vi "iRobot UART Read.vi"(8 "error in":errorcluster, 9 "timeout (ms)":i32=-1, 10 "Number of Bytes":u32, 11 "UART port in":T1) -> (0 "error out":errorcluster, 1 "UART Stream":u8[](array[numeric]), 2 "Timed Out?":bool, 3 "UART port out":T1)   [LabVIEW 2015]
doc: "Read data from the UART receive buffer until <b>Number of Bytes</b> have been received, or until a timeout occurs. A negative timeout means wait indefinitely."
uses:
  iRobot UART Port Type.ctl
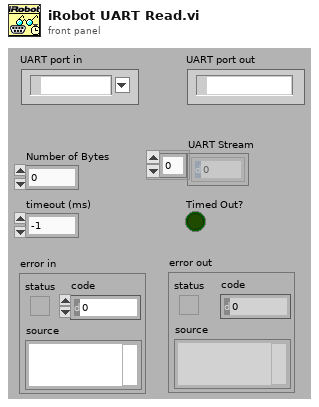
[diagram p1: front panel]
types:
  T1 = typedef "iRobot UART Port Type.ctl" = refnum<visa-resource-name>
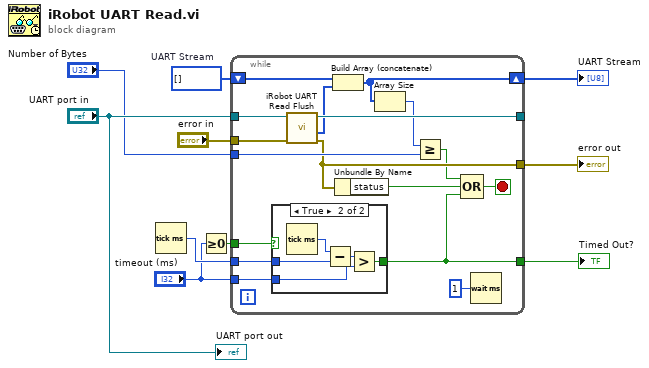
[diagram p0: block diagram]
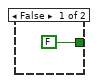
[diagram p2: hidden frame]
diagram:
  w1 = u8[] []  # UART Stream
  n1 = Tick Count (ms)() -> (millisecond timer value=w7:u32)
  n2 = Greater Or Equal To 0?(x="timeout (ms)") -> (x >= 0?=w5:bool)
  n3 = while {
    shift-right: [w13] -> w9
    shift-left: w1 -> [w15]
    tunnel: "UART port in" -> [w27]
    tunnel: [w26] -> _
    tunnel: "Number of Bytes" -> [w25]
    tunnel: w7 -> [w24]
    tunnel: "timeout (ms)" -> [w23]
    tunnel: [w18] -> w6
    tunnel: w5 -> [w21]
    tunnel: "error in" -> [w20]
    tunnel: [w17] -> w2
    stop <- w19 stop-if-true
    n4 = case shown="True" w21 {
      tunnel: w24 -> [_ w33]
      tunnel: w23 -> [_ w30]
      tunnel: [FALSE w29] -> w18
      frame False {
      }
      frame True {
        n5 = Tick Count (ms)() -> (millisecond timer value=w32:u32)
        n6 = Subtract(x=w32, y=w33) -> (x-y=w31:u32)
        n7 = Greater?(x=w31, y=w30) -> (0:w29:bool)
      }
    }
    n8 = call "iRobot UART Read Flush.vi"("error in"=w20, "UART port in"=w27) -> ("error out"=w17:errorcluster, "data"=w14:u8[], "UART port out"=w26:T1)  [unwired: 7 out]
    n9 = Build Array (concatenate)(w15, w14) -> (w13:u8[])
    n10 = Unbundle By Name(w17) -> ("status"=w12:bool)
    n11 = Array Size(array=w13) -> (size(s)=w16:i32)
    n12 = Greater Or Equal?(x=w16, y=w25) -> (x >= y?=w11:bool)
    n13 = Compound Arithmetic op=OR(w11, w12, w18) -> (w19:bool)
    n14 = Wait (ms)(milliseconds to wait=u32 1) -> ()  [unwired: 1 out]
  }
  "UART Stream" <- w9
  "Timed Out?" <- w6
  "error out" <- w2
  "UART port out" <- "UART port in"
